vi "Read Exported Data Location.vi"(8 "error in (no error)":errorcluster, 11 "Harmonics_CHP in":refnum<class "RxBN_CHP.lvclass">=refnum) -> (0 "error out":errorcluster, 2 "Exported Data Location":string, 3 "Harmonics_CHP out":refnum<class "RxBN_CHP.lvclass">)   [LabVIEW 2016, in "SeqAuto Evaluations.lvlib" / "RxBN_CHP.lvclass"]
uses:
  RxBN_CHP.lvclass
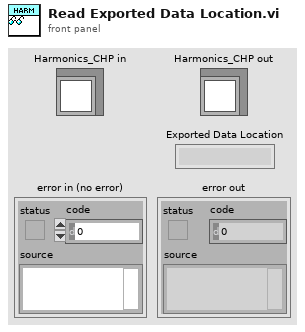
[diagram p1: front panel]
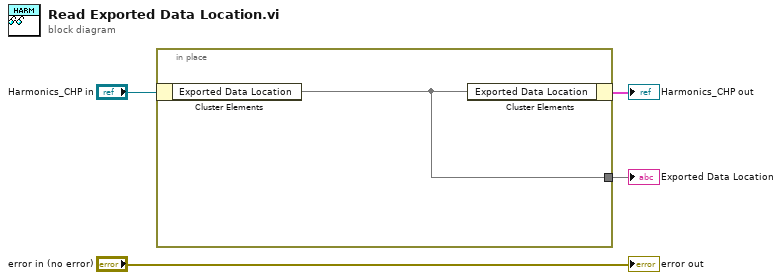
[diagram p0: block diagram]
diagram:
  n1 = in-place {
    in-place-border: [w5] -> w2
    n2 = in-place-cluster #1("Harmonics_CHP in") -> ("Exported Data Location"=w5)
    n3 = in-place-cluster #1("Exported Data Location"=w5) -> (→"Harmonics_CHP out":cluster{})
  }
  "Exported Data Location" <- w2
  "error out" <- "error in (no error)"
